vi "Disconnect.vi"(8 "error in (no error)":errorcluster, 11 "SolarSystems M266 Old in":refnum<class "SolarSystems M266 Old.lvclass">) -> (0 "error out":errorcluster, 3 "SolarSystems M266 Old out":refnum<class "SolarSystems M266 Old.lvclass">)   [LabVIEW 2014, in "SolarSystems M266 Old.lvclass"]
uses:
  SolarSystems M266 Old.lvclass
  SolarSystems M266 Old.lvclass/SolarSystems M266 Old.ctl
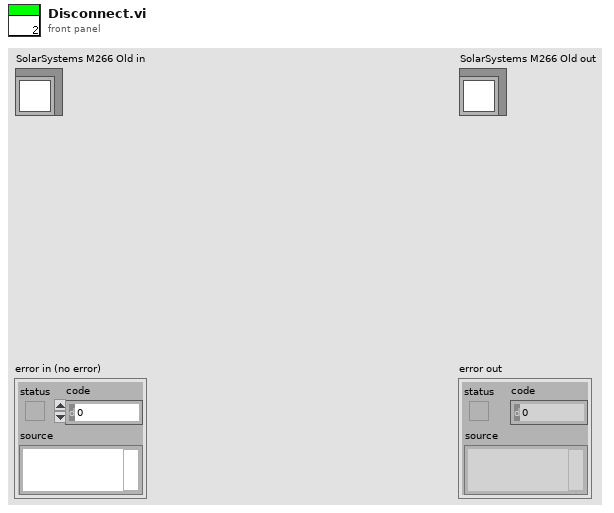
[diagram p1: front panel]
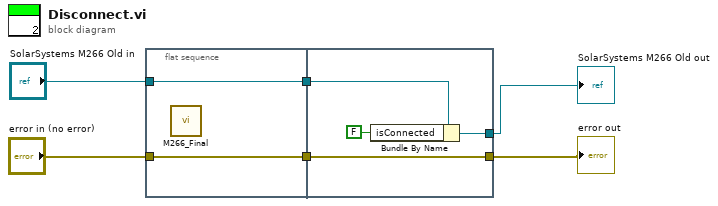
[diagram p0: block diagram]
diagram:
  n1 = flat-sequence {
    tunnel: "error in (no error)" -> [w7]
    tunnel: "SolarSystems M266 Old in" -> [w8]
    tunnel: [w8] -> w2
    tunnel: [w7] -> w1
    tunnel: [w11] -> w5
    tunnel: [w10] -> w3
    tunnel: w2 -> [w12]
    tunnel: w1 -> [w10]
    frame #0 {
      n2 = call "M266_Final.vi"() -> ()  [unwired: 1 in]
    }
    frame #1 {
      n3 = Bundle By Name(cluster=w12, "isConnected"=FALSE) -> (w11:refnum<class "SolarSystems M266 Old.lvclass">)
    }
  }
  "error out" <- w3
  "SolarSystems M266 Old out" <- w5
